vi "Get-start-path.vi"(8 "error in (no error)":errorcluster, 11 "SettingsFile in":refnum<class "SettingsFile.lvclass">) -> (0 "error out":errorcluster, 2 "File path":path, 3 "SettingsFile out":refnum<class "SettingsFile.lvclass">)   [LabVIEW 2013, in "SettingsFile.lvlib" / "SettingsFile.lvclass"]
uses:
  SettingsFile.lvclass
  SettingsFile.lvclass/SettingsFile.ctl
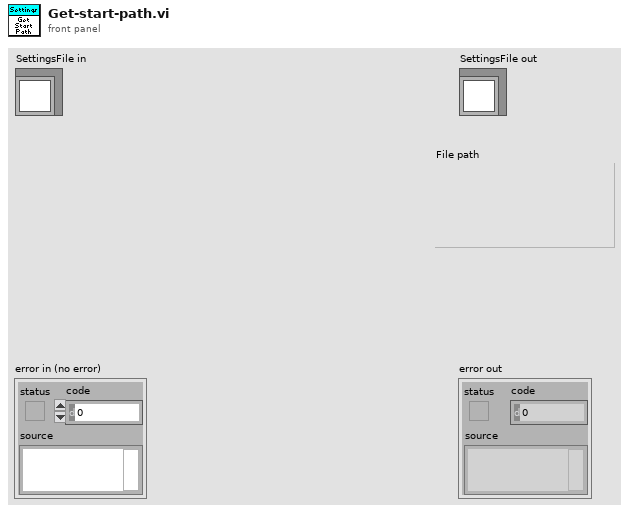
[diagram p1: front panel]
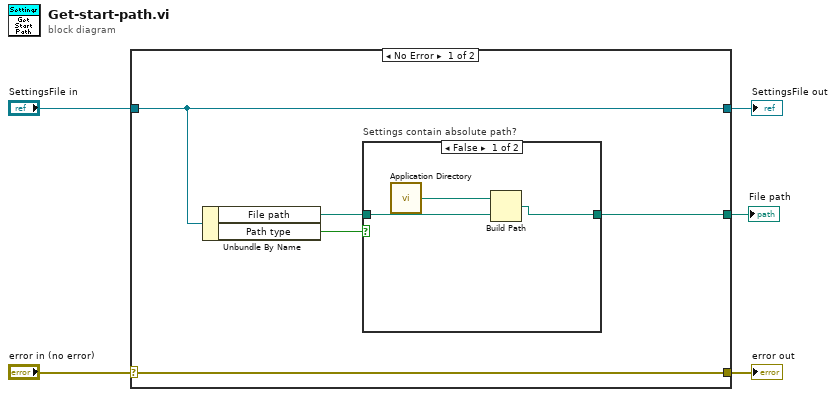
[diagram p0: block diagram]
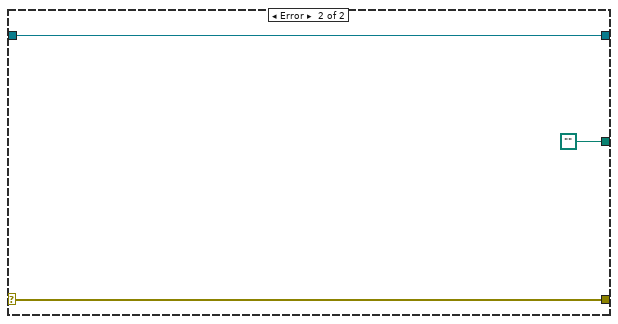
[diagram p3: hidden frame]
diagram:
  n1 = case shown="No Error" "error in (no error)" {
    selector: "error in (no error)" -> [w10 w17]
    tunnel: [w10 w17] -> w4
    tunnel: [w9 w16] -> w2
    tunnel: "SettingsFile in" -> [w9 w16]
    tunnel: [w6 path ""] -> w1
    frame No Error {
      n2 = Unbundle By Name(w9) -> ("File path"=w7:path, "Path type"=w8:bool)
      n3 = case "Settings contain absolute path?" shown="False" w8 {
        tunnel: w7 -> [w12 w14]
        tunnel: [w11 w14] -> w6
        frame False {
          n4 = call <vilib>:"Application Directory.vi"() -> ("Application Directory"=w13:path)
          n5 = Build Path(base path=w13, name or relative path=w12) -> (appended path=w11:path)
        }
        frame True {
        }
      }
    }
    frame Error {
    }
  }
  "error out" <- w4
  "SettingsFile out" <- w2
  "File path" <- w1
